vi "enqueue_pressure_auto_offset.vi"(0 "autoOffsetPsatQueue":refnum<queue>, 1 "# to average":dbl=100.0 format="%#_13g", 2 "Auto Offset":refnum<vi>, 3 "Pressure/Temperature/Mixture Properties":T1={"Line Densities\n[g/cm^3]"={"Vapor Line"=0.15445189986836314, "Liquid Line"=0.25755261741892205}, "Mixture Properties"={"Enthalpy"=195841526251804.2, "Quality [-]"=-10.825375459319764}, "Component PTs"={"Liquid Tank P"=3834985507386.06, "Liquid Tank T"=456.4106234658312, "Liquid Tank Sat P"=1736233577203.0627, "Liquid Tank Sat T"=492.17973224367375, "Separator P"=179910.46497250997, "Separator T"=-13120080.345725078, "Separator Sat P"=0.0, "Separator Sat T"=30.62899308837065, "Liquid Inlet P"=185261.09355383943, "Liquid Inlet T"=508.4593419640114, "Liquid Inlet Sat P"=12378986008470.418, "Liquid Inlet Sat T"=31.430570229281372, "Vapor Tank P"=108956.35947325415, "Vapor Tank T"=-10372083.904135285, "Vapor Tank Sat P"=0.0, "Vapor Tank Sat T"=16.912041354361705, "Vapor Inlet P"=379651.1166364239, "Vapor Inlet T"=381.53210552887515, "Vapor Inlet Sat P"=102884868683.01198, "Vapor Inlet Sat T"=51.054688909951395, "Test Section P"=44976.833741485905, "Test Section T"=-16719245.882515587, "Test Section Sat P"=0.0, "Test Section Sat T"=-7.288297090299707, "Upper Dev Section P"=0.0, "Upper Dev Section T"=0.0, "Upper Dev Section Sat P"=0.0, "Upper Dev Section Sat T"=0.0, "Lower Dev Section P"=0.0, "Lower Dev Section T"=0.0, "Lower Dev Section Sat P"=0.0, "Lower Dev Section Sat T"=0.0}, "Ambient Pressure [Pa]"=0.0, "Mixing Tee"={"Venturi dP"=0.0, "PGminiPressure"=0.0, "PGminiTemperature"=0.0}}, 4 "Auto Offset ProgressBar":refnum<vi>) -> ()   [LabVIEW 2017]
uses:
  pressure_temp_mixture.ctl
panel:
  # "Saturation\nPressure [Pa]"
  # "Saturation\nTemperature [C]"
  # "Pressure [Pa]"
  # "Temperature [C]"
  # "Liquid Tank"
  # "Separator"
  # "Liquid Inlet"
  # "Vapor Tank"
  # "Vapor Inlet"
  # "Test Section"
  # "Upper Dev Section"
  # "Lower Dev Section"
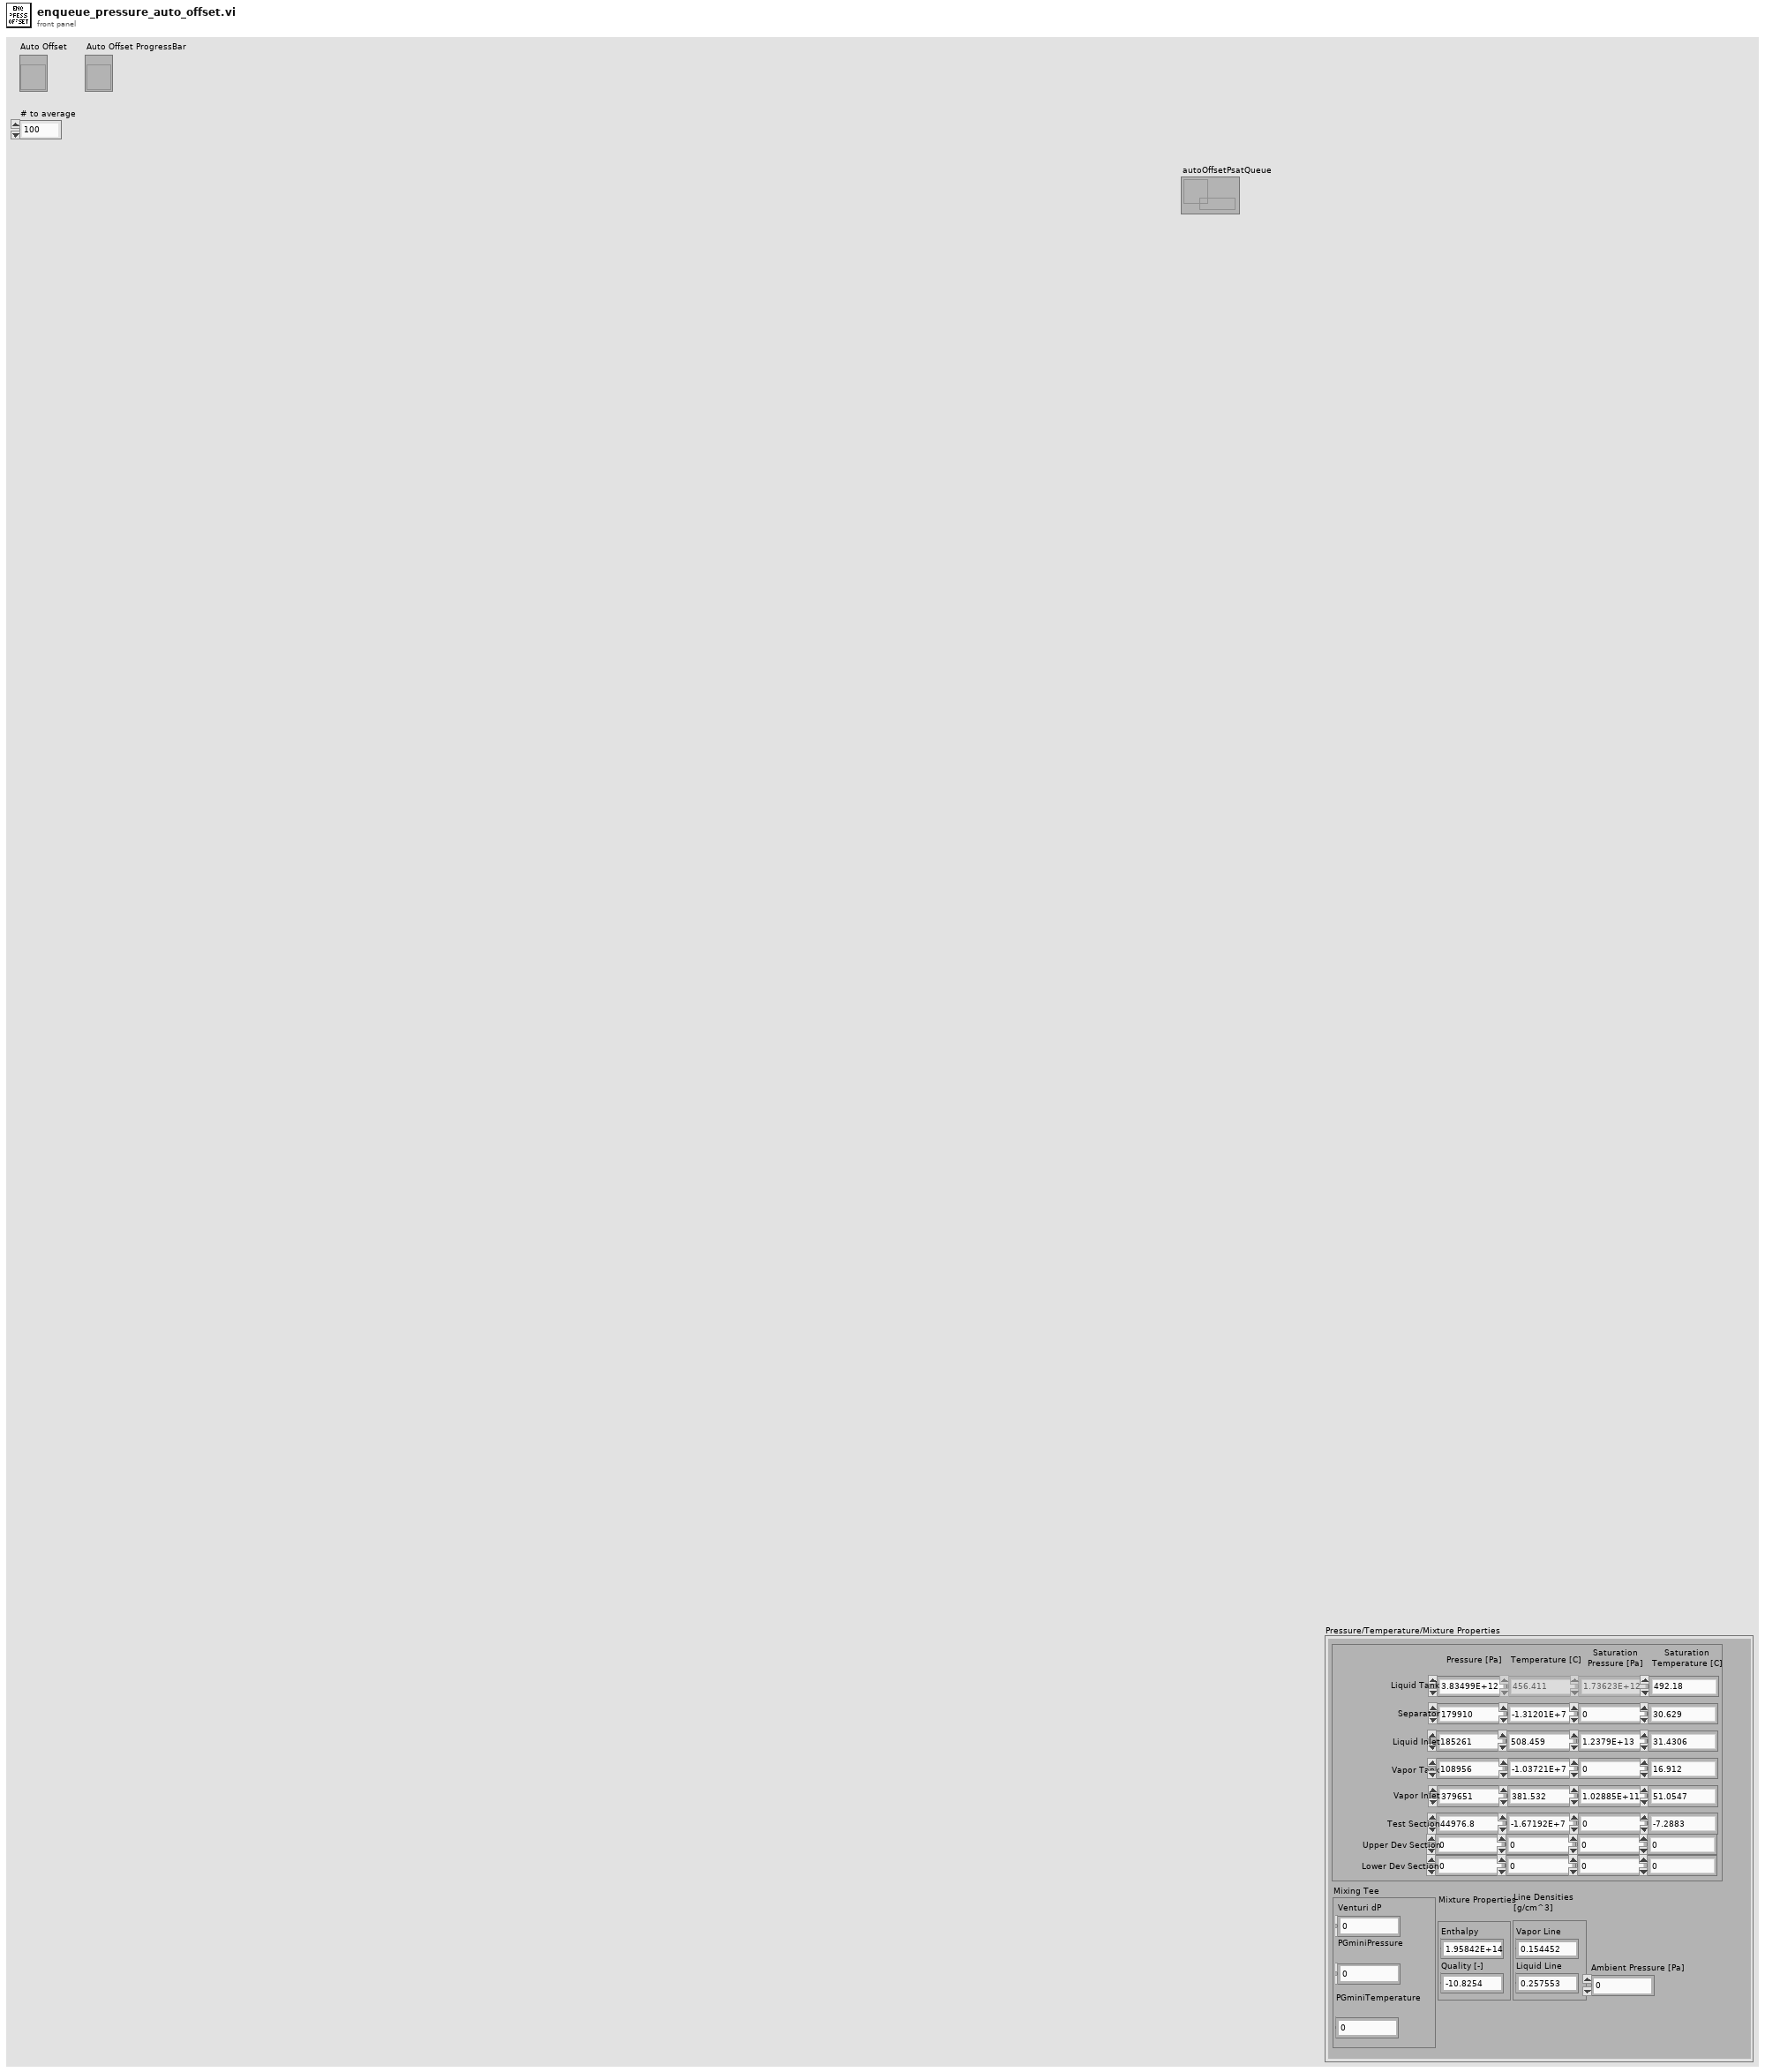
[diagram p1: front panel]
types:
  T1 = typedef "pressure_temp_mixture.ctl" = cluster{"Line Densities\n[g/cm^3]":cluster{"Vapor Line":dbl, "Liquid Line":dbl}, "Mixture Properties":cluster{"Enthalpy":dbl, "Quality [-]":dbl}, "Component PTs":cluster{"Liquid Tank P":dbl, "Liquid Tank T":dbl, "Liquid Tank Sat P":dbl, "Liquid Tank Sat T":dbl, "Separator P":dbl, "Separator T":dbl, "Separator Sat P":dbl, "Separator Sat T":dbl, "Liquid Inlet P":dbl, "Liquid Inlet T":dbl, "Liquid Inlet Sat P":dbl, "Liquid Inlet Sat T":dbl, "Vapor Tank P":dbl, "Vapor Tank T":dbl, "Vapor Tank Sat P":dbl, "Vapor Tank Sat T":dbl, "Vapor Inlet P":dbl, "Vapor Inlet T":dbl, "Vapor Inlet Sat P":dbl, "Vapor Inlet Sat T":dbl, "Test Section P":dbl, "Test Section T":dbl, "Test Section Sat P":dbl, "Test Section Sat T":dbl, "Upper Dev Section P":dbl, "Upper Dev Section T":dbl, "Upper Dev Section Sat P":dbl, "Upper Dev Section Sat T":dbl, "Lower Dev Section P":dbl, "Lower Dev Section T":dbl, "Lower Dev Section Sat P":dbl, "Lower Dev Section Sat T":dbl}, "Ambient Pressure [Pa]":dbl, "Mixing Tee":cluster{"Venturi dP":dbl, "PGminiPressure":dbl, "PGminiTemperature":dbl}}
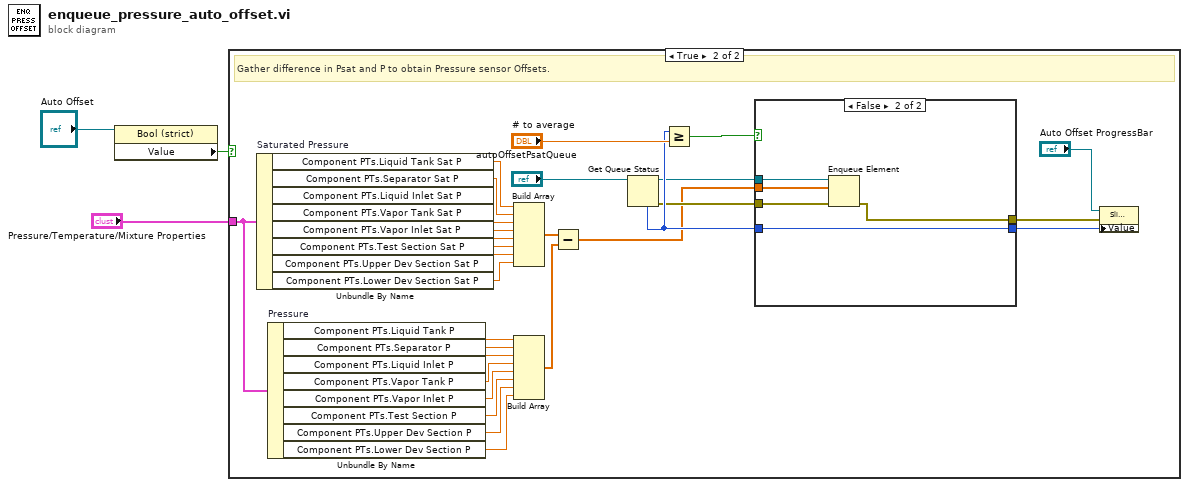
[diagram p0: block diagram]
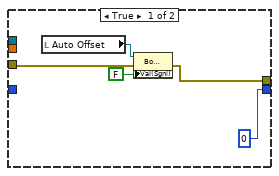
[diagram p3: hidden frame]
diagram:
  n1 = property class="Bool (strict)"(reference="Auto Offset") -> ("Value"=w1:bool)  [unwired: 1 in, 2 out]
  n2 = case shown="True" w1 {
    tunnel: "Pressure/Temperature/Mixture Properties" -> [_ w14]
    frame False {
    }
    frame True {
      # "Gather difference in Psat and P to obtain Pressure sensor Offsets."
      n3 = Unbundle By Name "Saturated Pressure"(w14) -> ("Component PTs.Liquid Tank Sat P"=w20:dbl, "Component PTs.Separator Sat P"=w21:dbl, "Component PTs.Liquid Inlet Sat P"=w22:dbl, "Component PTs.Vapor Tank Sat P"=w23:dbl, "Component PTs.Vapor Inlet Sat P"=w24:dbl, "Component PTs.Test Section Sat P"=w25:dbl, "Component PTs.Upper Dev Section Sat P"=w26:dbl, "Component PTs.Lower Dev Section Sat P"=w10:dbl)
      n4 = Unbundle By Name "Pressure"(w14) -> ("Component PTs.Liquid Tank P"=w32:dbl, "Component PTs.Separator P"=w31:dbl, "Component PTs.Liquid Inlet P"=w30:dbl, "Component PTs.Vapor Tank P"=w29:dbl, "Component PTs.Vapor Inlet P"=w28:dbl, "Component PTs.Test Section P"=w27:dbl, "Component PTs.Upper Dev Section P"=w13:dbl, "Component PTs.Lower Dev Section P"=w9:dbl)
      n5 = Build Array(w20, w21, w22, w23, w24, w25, w26, w10) -> (w19:dbl[])
      n6 = Build Array(w32, w31, w30, w29, w28, w27, w13, w9) -> (w18:dbl[])
      n7 = Subtract(x=w19, y=w18) -> (x-y=w5:dbl[])
      n8 = Get Queue Status(queue="autoOffsetPsatQueue") -> (queue out=w7:refnum<queue>, error out=w6:errorcluster, # elements in queue=w15:i32)  [unwired: 2 in, 5 out]
      n9 = Greater Or Equal?(x=w15, y="# to average") -> (x >= y?=w17:bool)
      n10 = case shown="False" w17 {
        tunnel: w15 -> [_ w42]
        tunnel: [u32 0 ("Auto Offset Progress") w42] -> w11
        tunnel: w7 -> [_ w41]
        tunnel: w6 -> [w34 w40]
        tunnel: w5 -> [_ w39]
        tunnel: [w33 w38] -> w4
        frame True {
          n11 = local read "Auto Offset"() -> (w36:refnum<vi>)
          n12 = property class="Bool (strict)"(reference=w36, error in=w34, "Val(Sgnl)"=FALSE) -> (error out=w33:errorcluster)  [unwired: 1 out]
        }
        frame False {
          n13 = Enqueue Element(queue=w41, element=w39, error in (no error)=w40) -> (error out=w38:errorcluster)  [unwired: 1 in, 2 out]
        }
      }
      n14 = property class="Slide (strict)"(reference="Auto Offset ProgressBar", error in=w4, "Value"=w11) -> ()  [unwired: 2 out]
    }
  }
